vi "Temp2.vi"(9 "c":u32, 10 "b":u32, 11 "a":u32) -> (2 "Temp 2":u32)   [LabVIEW 2017, in "Crypto.lvlib" / "SHA-256.lvclass"]
uses:
  SHA-256.lvclass
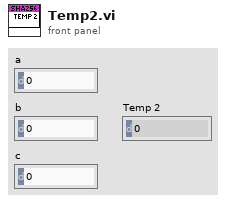
[diagram p1: front panel]
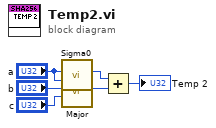
[diagram p0: block diagram]
diagram:
  n1 = call "Sigma0.vi"("Value"="a") -> ("Sigma 0"=w6:u32)  [unwired: 10 in]
  n2 = call "Major.vi"("c"="c", "b"="b", "a"="a") -> ("Major"=w5:u32)  [unwired: 8 in]
  n3 = Add(x=w6, y=w5) -> (x+y=→"Temp 2":u32)
